vi "Unix_Epoch_in_Labview.vi"() -> (0 "Unix epoch (seconds)":dbl=2082844800.0 format="%#.17g")   [LabVIEW 2021, in "Ring Buffer Strict Accessor.lvlib" / "Unix time epoch.lvlib"]
uses:
  Unix time epoch.lvlib
panel:
  out "Unix epoch":timestamp=timestamp(2082844800 s since 1904-01-01) format="%^< %H:%M:%S\n%m:%d:%Y>T"
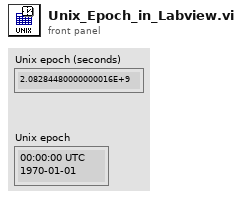
[diagram p1: front panel]
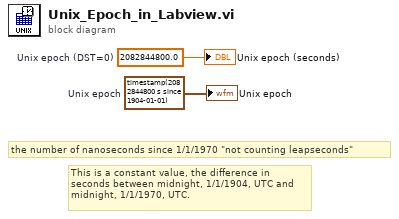
[diagram p0: block diagram]
diagram:
  w1 = timestamp(2082844800 s since 1904-01-01)  # Unix epoch
  w2 = 2082844800.0  # Unix epoch (DST=0)
  # "This is a constant value, the difference in seconds between midnight, 1/1/1904, UTC and midnight, 1/1/1970, UTC."
  # "the number of nanoseconds since 1/1/1970 \"not counting leapseconds\""
  "Unix epoch (seconds)" <- w2
  "Unix epoch" <- w1
